vi "RS_SMBV100A_CONVERT_DATASAT_2D_to_N1D.vi"(6 "2D DATA SAT":dbl[][](array[numeric])) -> (0 "GNSS_SatSkySortedMaxToMin":dbl[](array[numeric]), 1 "GNSS_SatSortedMaxToMin":dbl[](array[numeric]), 3 "GNSS_SatSkySortedMinToMax":dbl[](array[numeric]), 4 "GNSS_SatSortedMinToMax":dbl[](array[numeric]), 5 "GNSS_TimeSortedMaxToMin":dbl[](array[numeric]), 8 "GNSS_TimeSortedMinToMax":dbl[](array[numeric]))   [LabVIEW 2018]
uses:
  <userlib>/_OpenG.lib/array/array.llb/Sort 2D Array (DBL)__ogtk.vi
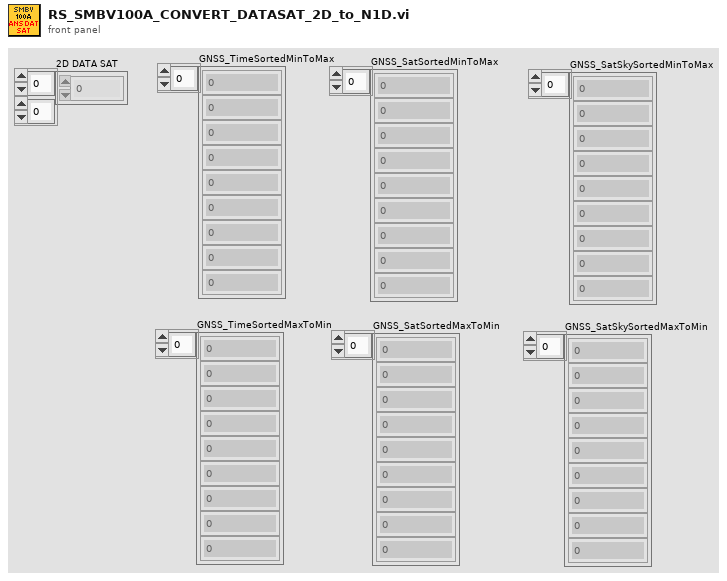
[diagram p1: front panel]
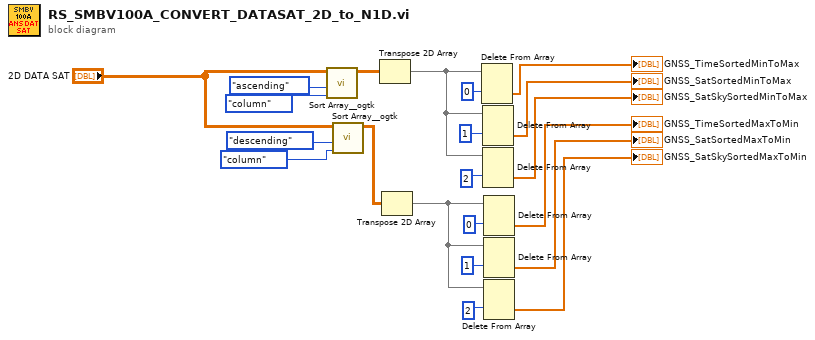
[diagram p0: block diagram]
diagram:
  n1 = call-poly <userlib>:"Sort Array__ogtk.vi"("Sort By in"=enum16{"row", "column"}."column", "Order"=enum16{"ascending", "descending"}."ascending", "Array in"="2D DATA SAT") -> ("Sorted Array out"=w17:dbl[][])  [unwired: 5 in, 3 out]
  n2 = call-poly <userlib>:"Sort Array__ogtk.vi"("Sort By in"=enum16{"row", "column"}."column", "Order"=enum16{"ascending", "descending"}."descending", "Array in"="2D DATA SAT") -> ("Sorted Array out"=w8:dbl[][])  [unwired: 5 in, 3 out]
  n3 = Transpose 2D Array(2D array=w17) -> (transposed array=w13:dbl[][])
  n4 = Transpose 2D Array(2D array=w8) -> (transposed array=w9:dbl[][])
  n5 = Delete From Array(array=w13, index (row)=0) -> (deleted portion=→"GNSS_TimeSortedMinToMax":dbl[])  [unwired: 2 in, 1 out]
  n6 = Delete From Array(array=w13, index (row)=1) -> (deleted portion=→"GNSS_SatSortedMinToMax":dbl[])  [unwired: 2 in, 1 out]
  n7 = Delete From Array(array=w13, index (row)=2) -> (deleted portion=→"GNSS_SatSkySortedMinToMax":dbl[])  [unwired: 2 in, 1 out]
  n8 = Delete From Array(array=w9, index (row)=0) -> (deleted portion=→"GNSS_TimeSortedMaxToMin":dbl[])  [unwired: 2 in, 1 out]
  n9 = Delete From Array(array=w9, index (row)=1) -> (deleted portion=→"GNSS_SatSortedMaxToMin":dbl[])  [unwired: 2 in, 1 out]
  n10 = Delete From Array(array=w9, index (row)=2) -> (deleted portion=→"GNSS_SatSkySortedMaxToMin":dbl[])  [unwired: 2 in, 1 out]
